vi "Configure Tx Bandwidth Offset.vi"(7 "Tx Bandwidth Offset (0)":i32, 8 "error in (no error)":errorcluster, 9 "CC (1)":T1=1, 10 "Instance (1)":T2=1, 11 "VISA resource name":refnum<visa-resource-name>) -> (0 "error out":errorcluster, 3 "VISA resource name out":refnum<visa-resource-name>)   [LabVIEW 2020, in "Rohde&Schwarz CMWXP NR FR1 Measurement.lvlib"]
doc: "Specifies the offset to carrier (TxBW offset) of carrier <no>.\n\nAttribute:\nRSCMWXPNRFR1M_ATTR_TX_BANDWIDTH_OFFSET\n\nRemote-control command:\nCONFigure:NRSub:MEAS<i>[:CC<no>]:TXBWidth:OFFSet"
uses:
  <instrlib>/Rohde&Schwarz CMWXP NR FR1 Measurement/Rohde&Schwarz CMWXP NR FR1 Measurement.lvlib
  <instrlib>/Rohde&Schwarz CMWXP NR FR1 Measurement/Private/_Instance.ctl
  <instrlib>/Rohde&Schwarz CMWXP NR FR1 Measurement/Private/_Carrier Component.ctl
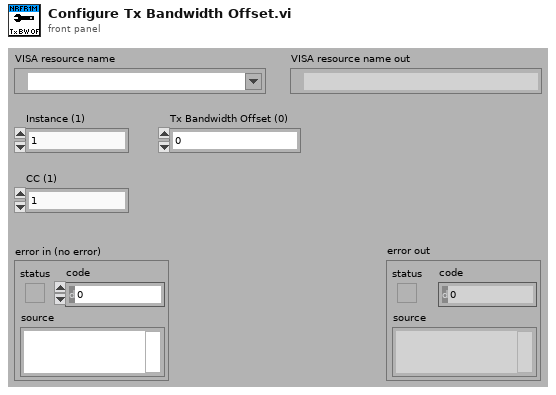
[diagram p1: front panel]
types:
  T1 = typedef "Rohde&Schwarz CMWXP NR FR1 Measurement.lvlib/_Carrier Component.ctl" = i32
  T2 = typedef "Rohde&Schwarz CMWXP NR FR1 Measurement.lvlib/_Instance.ctl" = i32
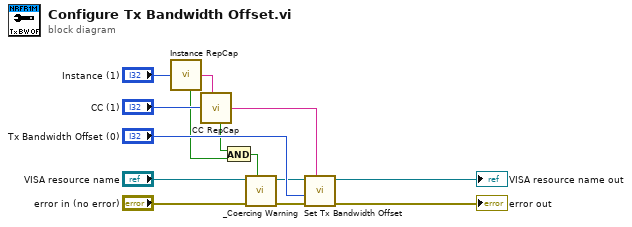
[diagram p0: block diagram]
diagram:
  n1 = call <instrlib>:"Instance RepCap.vi"("Instance In"="Instance (1)") -> ("In Range?"=w2:bool, "RepCap Identifier Out"=w11:string)  [unwired: 1 in]
  n2 = call <instrlib>:"CC RepCap.vi"("CC In"="CC (1)", "RepCap String In (\"\")"=w11) -> ("In Range?"=w1:bool, "RepCap Identifier Out"=w8:string)
  n3 = And(x=w1, y=w2) -> (x .and. y?=w3:bool)
  n4 = call <instrlib>:"_Coercing Warning.vi"("In Range?"=w3, "error in (no error)"="error in (no error)", "VISA resource name"="VISA resource name") -> ("error out"=w5:errorcluster, "VISA resource name out"=w4:refnum<visa-resource-name>)  [unwired: 7 in]
  n5 = call "Set Tx Bandwidth Offset"("Repeated Capabilities"=w8, "error in (no error)"=w5, "Tx Bandwidth Offset (0)"="Tx Bandwidth Offset (0)", "instrument handle"=w4) -> ("error out"=→"error out":errorcluster, "instrument handle out"=→"VISA resource name out":refnum<visa-resource-name>)  [unwired: 6 in]
